vi "Test Serialize Numbers.vi"(8 "error in (no error)":errorcluster) -> (0 "error out":errorcluster)   [LabVIEW 2013]
uses:
  <vilib>/addons/_JKI Toolkits/Caraya/classes/Test/Test.lvclass
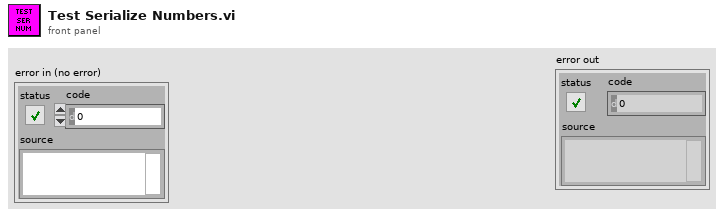
[diagram p1: front panel]
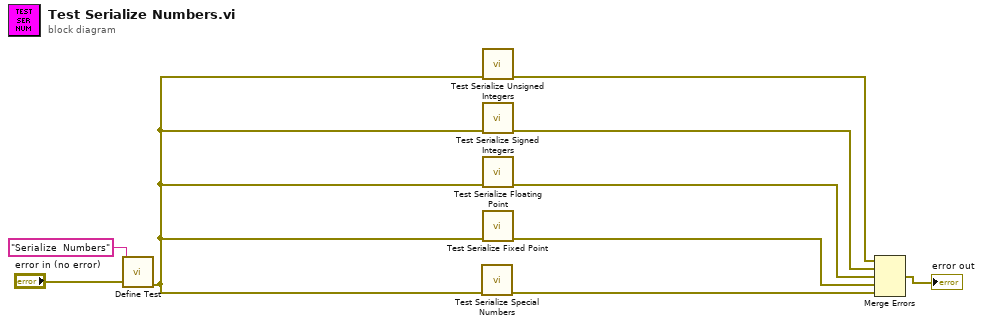
[diagram p0: block diagram]
diagram:
  n1 = call <vilib>:"Define Test.vi"("error in (no error)"="error in (no error)", "Label (VI Title)"="Serialize  Numbers") -> ("error out"=w6:errorcluster)  [unwired: 9 in]
  n2 = call "Test Serialize Special Numbers.vi"("error in (no error)"=w6) -> ("error out"=w1:errorcluster)  [unwired: 10 in]
  n3 = call "Test Serialize Unsigned Integers.vi"("error in (no error)"=w6) -> ("error out"=w5:errorcluster)  [unwired: 10 in]
  n4 = call "Test Serialize Signed Integers.vi"("error in (no error)"=w6) -> ("error out"=w4:errorcluster)  [unwired: 10 in]
  n5 = call "Test Serialize Floating Point.vi"("error in (no error)"=w6) -> ("error out"=w3:errorcluster)  [unwired: 10 in]
  n6 = call "Test Serialize Fixed Point.vi"("error in (no error)"=w6) -> ("error out"=w2:errorcluster)  [unwired: 10 in]
  n7 = Merge Errors(w5, w4, w3, w2, w1) -> (→"error out":errorcluster)
